vi "Set Segmenting Specification (Default).vi"(5 "Segment File on Trigger (T)":bool=TRUE, 7 "Max Instances (-1: Infinite)":i32=-1, 8 "error in (no error)":errorcluster, 11 "Data Logging Specification Ref in":T1) -> (0 "error out":errorcluster, 3 "Data Logging Specification Ref out":T1)   [LabVIEW 2020, in "NI_VS Data Logging API.lvlib"]
doc: "Specifies how to segment the log files created during the data logging session. You can segment log files according to time or size limits, or when a start trigger occurs. When the segmenting condition is met, this VI saves and closes the current log file and continues logging data in a new file.\n\nSelect the Default instance of this VI if you do not want to segment log files based on time or size, but do want the option to segment on a start trigger.\n\nYou must manually select the polymorphic instance to use."
uses:
  <vilib>/NI VeriStand/Execution/DataLogging/NI_VS Data Logging API.lvlib
  <vilib>/NI VeriStand/Execution/DataLogging/DataLoggingSpecification Ref.ctl
  NationalInstruments.VeriStand.ClientAPI
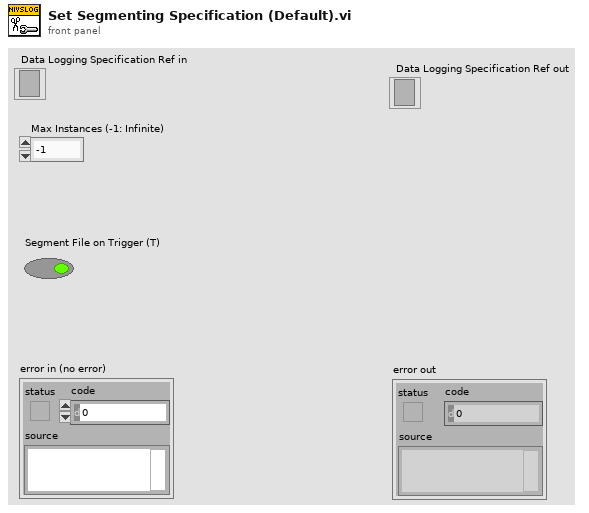
[diagram p1: front panel]
types:
  T1 = typedef "NI_VS Data Logging API.lvlib/DataLoggingSpecification Ref.ctl" = refnum<k24>
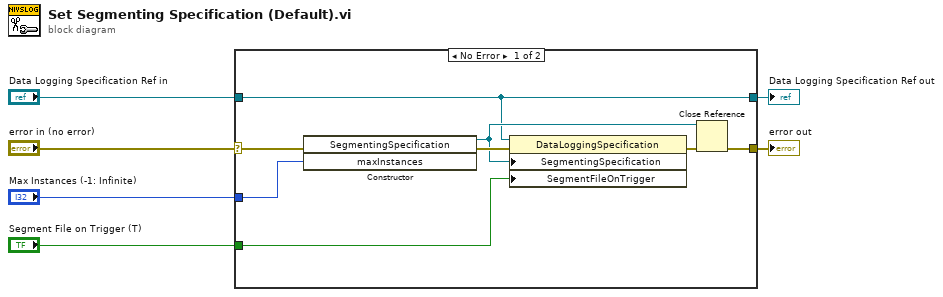
[diagram p0: block diagram]
diagram:
  n1 = case shown="No Error" "error in (no error)" {
    selector: "error in (no error)" -> [w14 w16]
    tunnel: [w10 w16] -> w5
    tunnel: [w8 w15] -> w4
    tunnel: "Data Logging Specification Ref in" -> [w8 w15]
    tunnel: "Max Instances (-1: Infinite)" -> [w13 _]
    tunnel: "Segment File on Trigger (T)" -> [w7 _]
    frame No Error {
      n2 = constructor class="SegmentingSpecification"(error in=w14, "maxInstances"=w13) -> (reference out=w9:refnum<k24>, error out=w12:errorcluster)  [unwired: 2 in, 2 out]
      n3 = property class="DataLoggingSpecification"(reference=w8, error in=w12, "SegmentingSpecification"=w9, "SegmentFileOnTrigger"=w7) -> (error out=w11:errorcluster)  [unwired: 1 out]
      n4 = Close Reference(reference=w9, error in (no error)=w11) -> (error out=w10:errorcluster)
    }
    frame Error {
    }
  }
  "error out" <- w5
  "Data Logging Specification Ref out" <- w4
